vi "ARRAY1.vi"(10 "Numeric 2":dbl, 11 "Numeric":dbl) -> (3 "Array 2":dbl[][](array[numeric]))   [LabVIEW 2018]
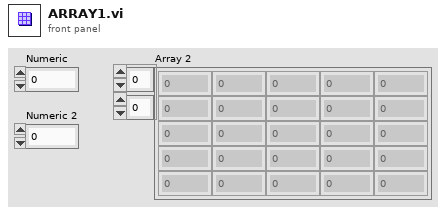
[diagram p1: front panel]
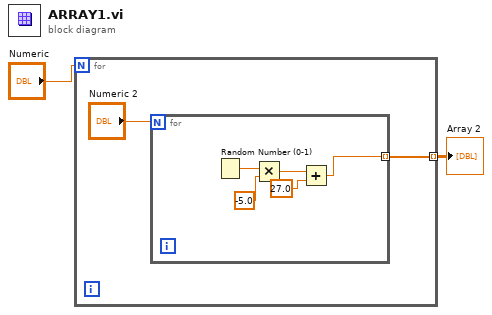
[diagram p0: block diagram]
diagram:
  n1 = for {
    N: "Numeric" -> [_]
    tunnel: [w3] -> w2 mode=indexing
    n2 = for {
      N: "Numeric 2" -> [_]
      tunnel: [w5] -> w3 mode=indexing
      n3 = Random Number (0-1)() -> (number: 0 to 1=w9:dbl)
      n4 = Multiply(x=w9, y=-5.0) -> (x*y=w7:dbl)
      n5 = Add(x=w7, y=27.0) -> (x+y=w5:dbl)
    }
  }
  "Array 2" <- w2
